vi "level_probe.vi"(5 "Run VI":bool, 6 "Set # of Turns Open (Man)":dbl, 7 "Target Level (Auto)":dbl format="%.2f", 8 "stop":bool, 9 "Mode":enum32{"AUTOMATIC", "MANUAL"}(radio)=enum."MANUAL", 10 "position":refnum<vi>, 11 "level":refnum<vi>) -> ()   [LabVIEW 2019]
uses:
  <vilib>/numeric/Random Number (Range) DBL.vi
  <vilib>/Utility/config.llb/Read Key (String).vi
  <vilib>/Utility/config.llb/Read Key (Path).vi
  <vilib>/Utility/file.llb/Read Delimited Spreadsheet (DBL).vi
  <vilib>/Utility/file.llb/Write Delimited Spreadsheet (DBL).vi
  subvi_motor/global_motor.vi
  <vilib>/addons/control/pid/NI_PID_autopid.lvlib
  <vilib>/Utility/config.llb/NI_LVConfig.lvlib
panel:
  out "read buffer":string
  in  "Mode 2":enum32{"Continuous", "Sample and Hold"}(radio)
  in  "Motor Enabled":bool=TRUE
  out "levelbuffer":string
  out "Level":dbl(slide) scale=0.0..100.0
  in  "Save PID gains":bool
  in  "Load PID gains":bool
  in  "Recalibrate":bool
  in  "Current Position":dbl
  out "Motor Connected":bool
  in  "Enable Advanced Controls":bool
  in  "Log Data?":bool
  out "maxsteps":dbl
  out "minsteps":dbl
  in  "Min Open (Auto)":dbl=0.25
  in  "Max Open (Auto)":dbl=0.75
  out "Level":dynamicdata(graph)
  out "Error":dynamicdata(graph)
  in  "PID gains":T1={"proportional gain (Kc)"=10.0, "integral time (Ti, min)"=0.002, "derivative time (Td, min)"=0.2} {"derivative time (Td, min)" format="%.3f"; "integral time (Ti, min)" format="%.3f"; "proportional gain (Kc)" format="%.3f"}
  out "Valve Position":dynamicdata(graph)
  out "# of Turns Open":dbl
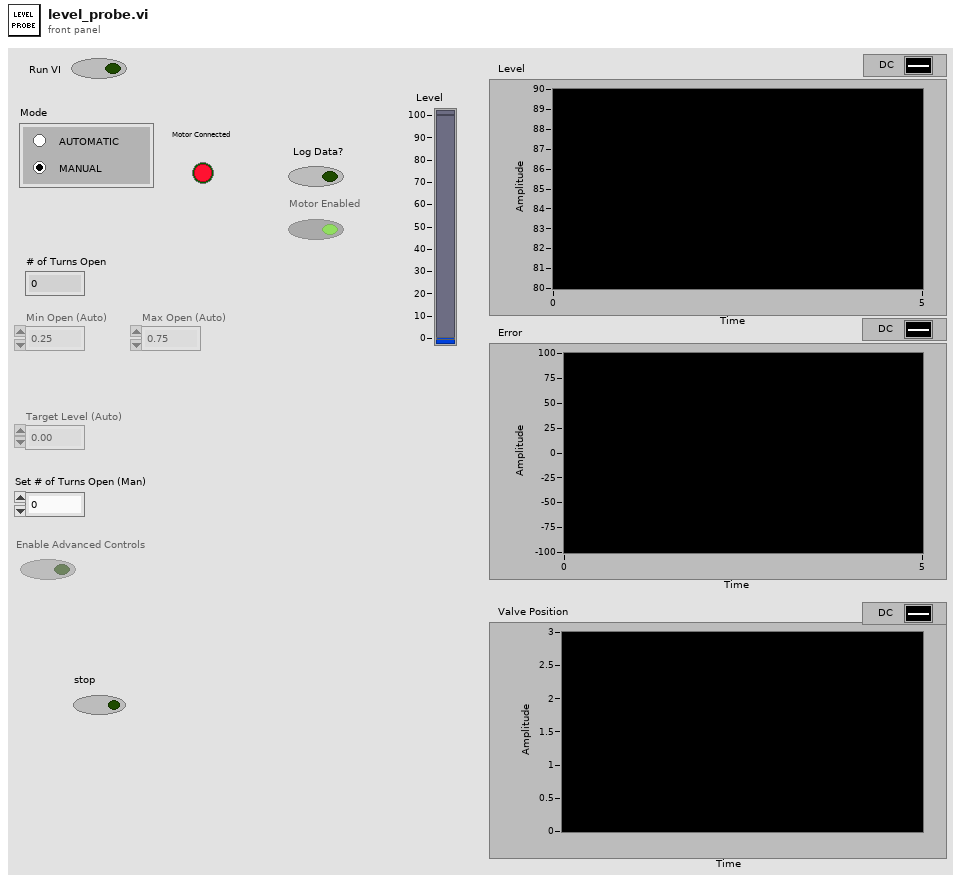
[diagram p1: front panel]
types:
  T1 = cluster{"proportional gain (Kc)":dbl, "integral time (Ti, min)":dbl, "derivative time (Td, min)":dbl}
  T2 = enum16{"open", "replace", "create", "open or create", "replace or create", "replace or create with confirmation"}
  T3 = enum8{"Enabled", "Disabled", "Disabled and Grayed Out"}
  T4 = typedef "NI_LVConfig.lvlib/Config Data RefNum.ctl" = refnum<k1>
  T5 = cluster{"first row[0]":dbl, "first row[1]":dbl, "first row[2]":dbl, "first row[3]":dbl, "first row[4]":dbl, "first row[5]":dbl, "first row[6]":dbl, "first row[7]":dbl, "first row[8]":dbl}
  T6 = cluster{"first row[0]":dbl, "first row[1]":dbl, "first row[2]":dbl}
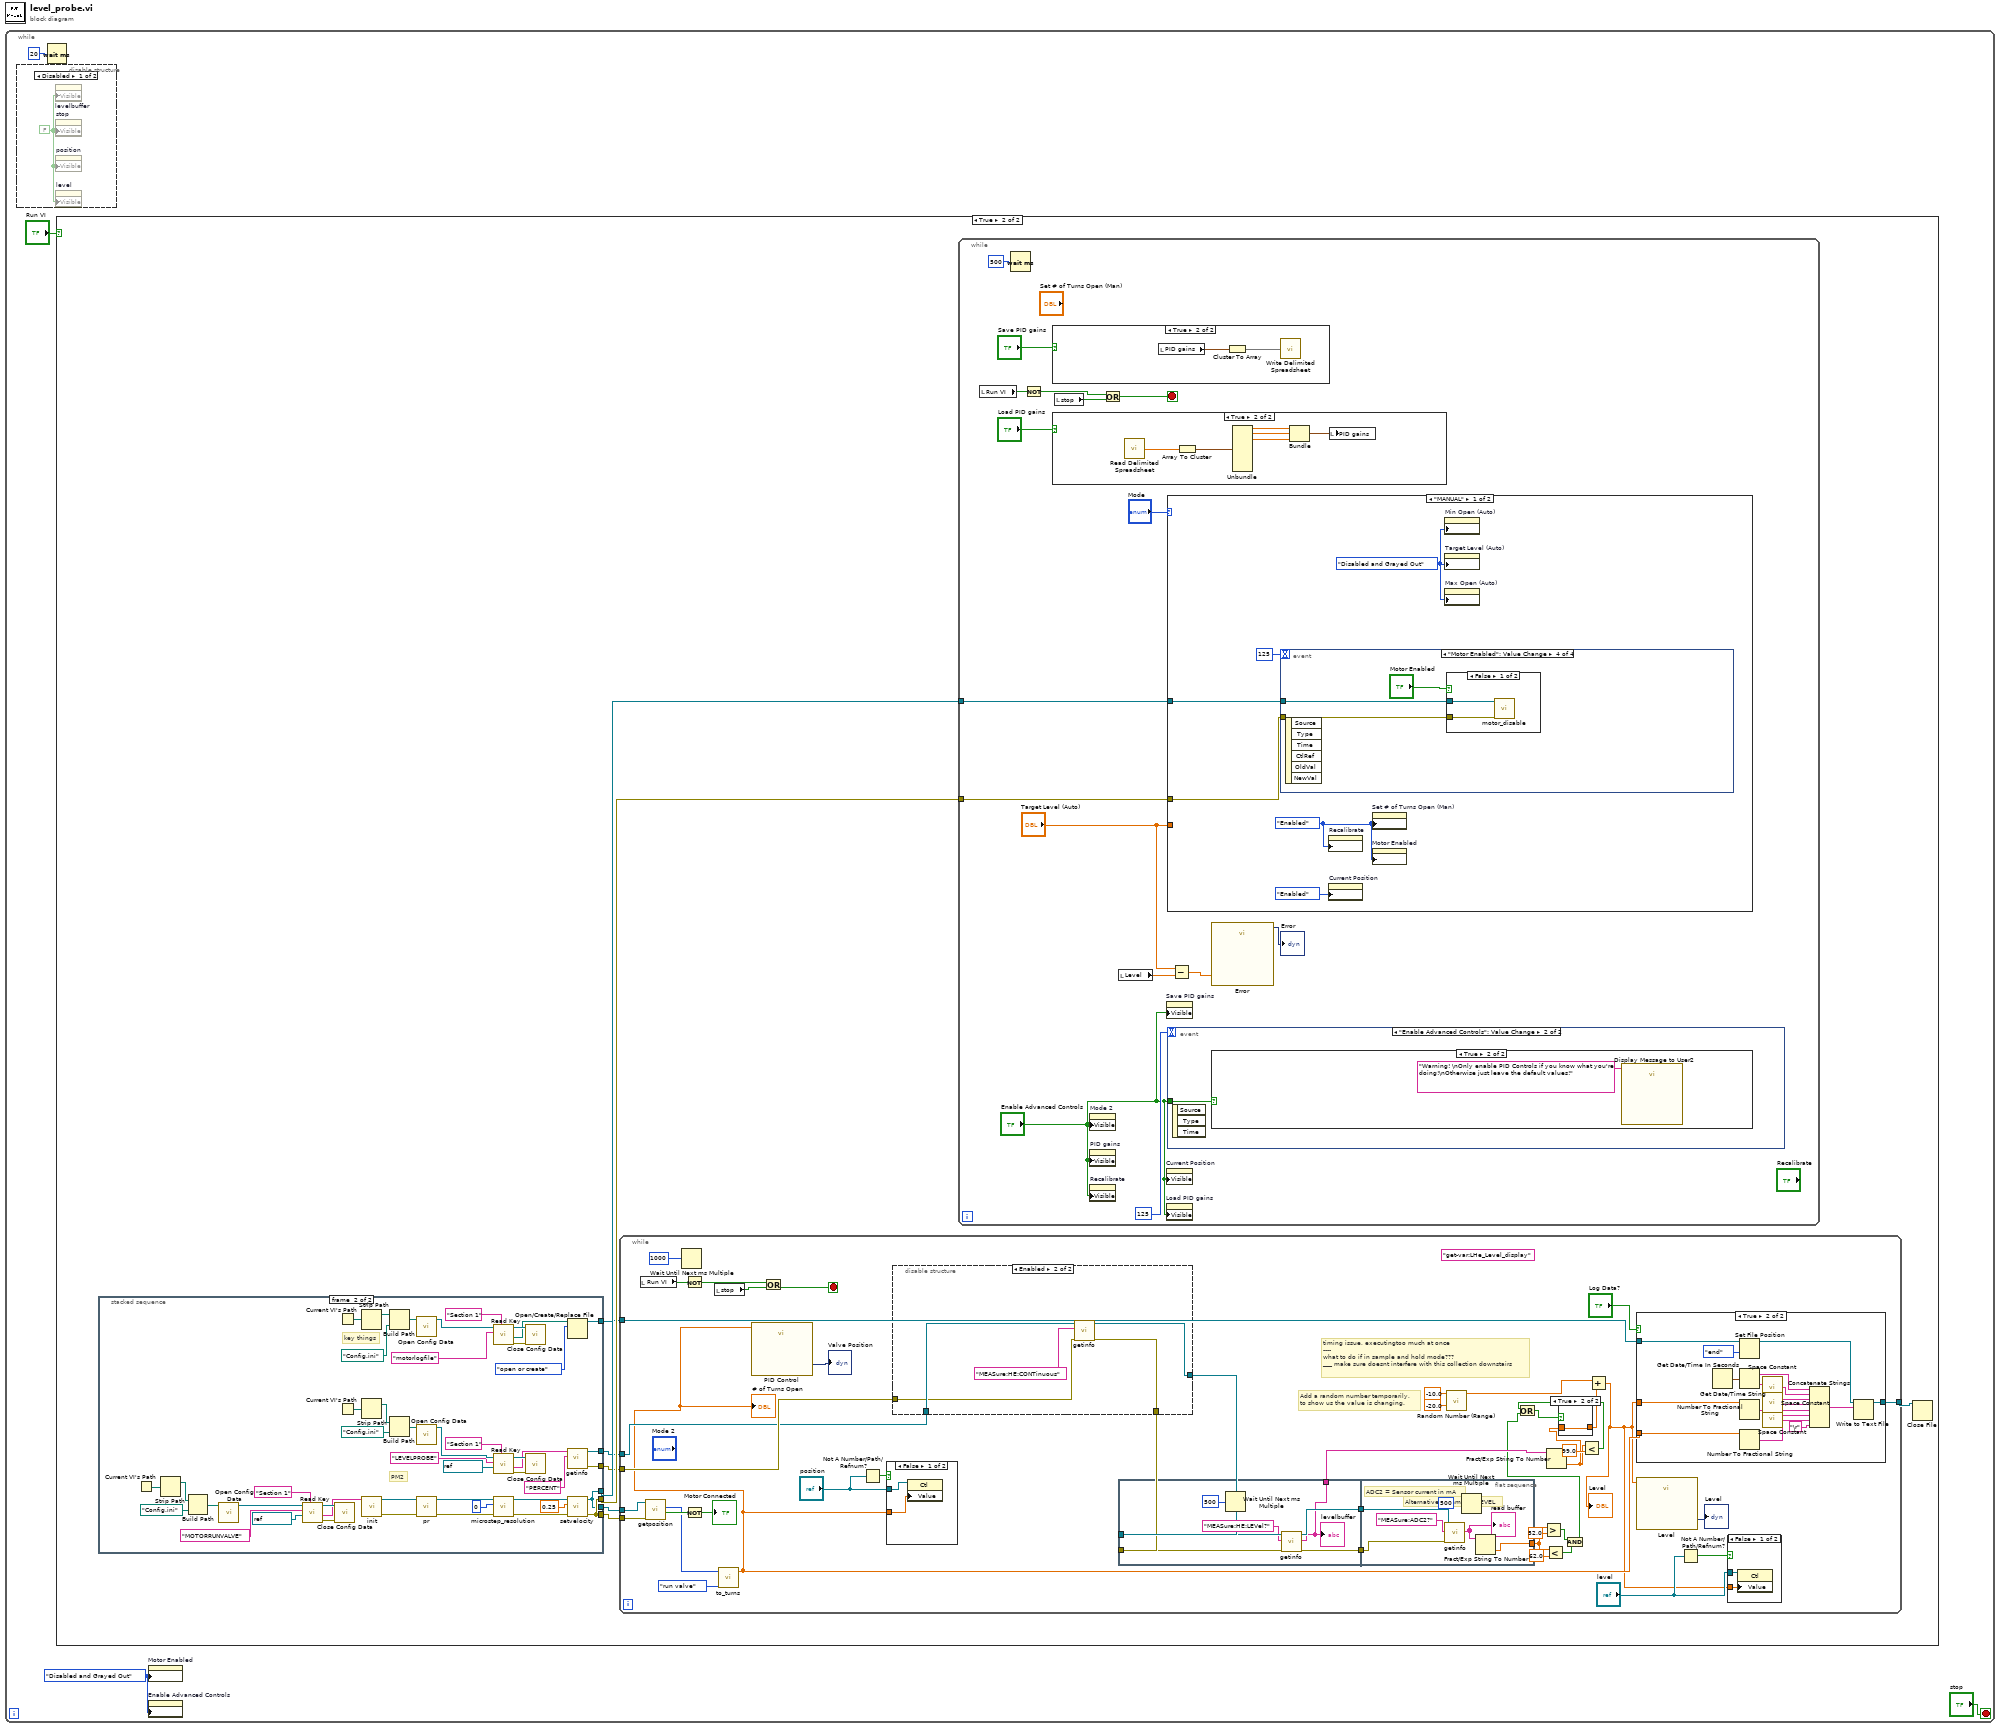
[diagram p0: block diagram]
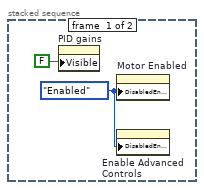
[diagram p4: hidden frame]
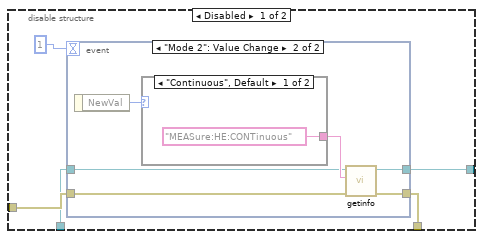
[diagram p5: hidden frame]
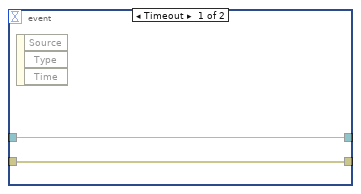
[diagram p6: hidden frame]
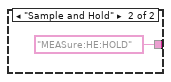
[diagram p7: hidden frame]
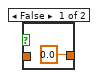
[diagram p10: hidden frame]
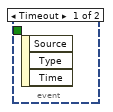
[diagram p12: hidden frame]
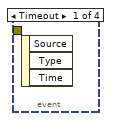
[diagram p16: hidden frame]
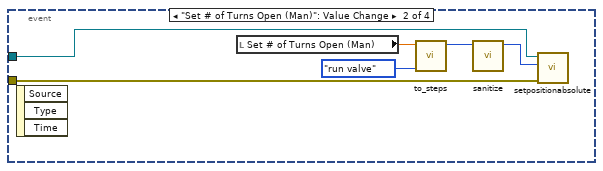
[diagram p17: hidden frame]
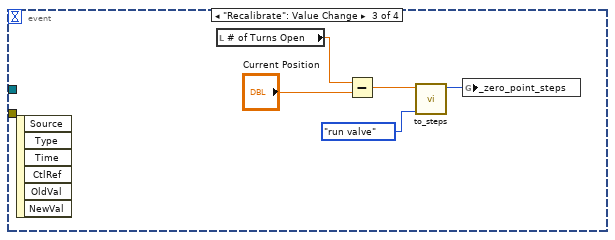
[diagram p18: hidden frame]
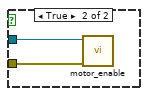
[diagram p19: hidden frame]
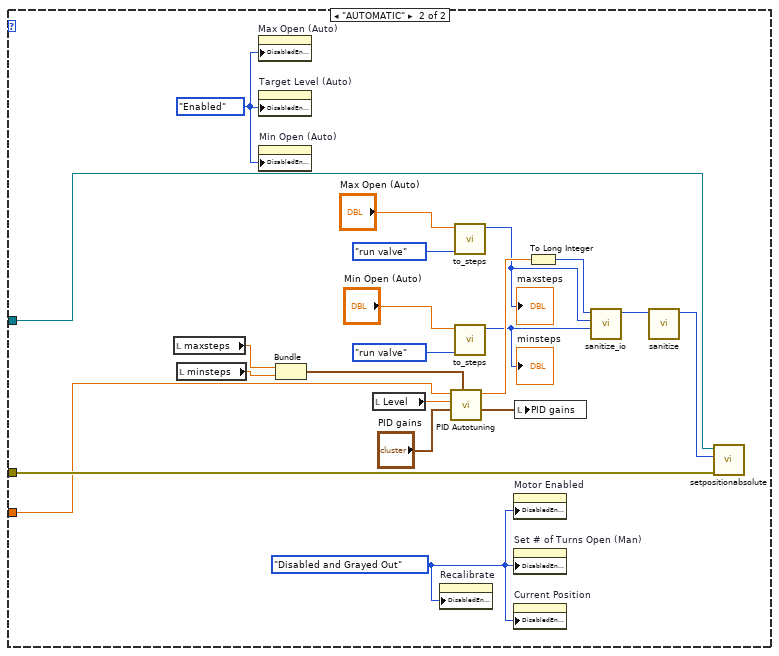
[diagram p20: hidden frame]
diagram:
  n1 = while {
    stop <- "stop" stop-if-true
    w1 = T3."Disabled and Grayed Out" ("Disabled")
    n2 = disable-structure shown="Disabled" {
      frame Disabled {
        w5 = FALSE ("Visible")
        n3 = property on="levelbuffer" class="Str"("Visible"=w5) -> ()  [unwired: 2 in, 2 out]
        n4 = property on="stop" class="Bool (strict)"("Visible"=w5) -> ()  [unwired: 2 in, 2 out]
        n5 = property on="position" class="LVObjRef (strict)"("Visible"=w5) -> ()  [unwired: 2 in, 2 out]
        n6 = property on="level" class="LVObjRef (strict)"("Visible"=w5) -> ()  [unwired: 2 in, 2 out]
      }
      frame Enabled {
      }
    }
    n7 = Wait (ms)(milliseconds to wait=u32 20) -> ()  [unwired: 1 out]
    n8 = case shown="True" "Run VI" {
      frame False {
      }
      frame True {
        n9 = stacked-sequence {
          tunnel: [_ w61] -> w13
          tunnel: [_ w61] -> w12
          tunnel: [_ w60] -> w11
          tunnel: [_ w60] -> w10
          tunnel: [_ w55] -> w9
          tunnel: [_ w54] -> w8
          tunnel: [_ w53] -> w7
          frame #0 {
            w14 = T3."Enabled" ("Disabled")
            n10 = property on="PID gains" class="Clust (strict)"("Visible"=FALSE) -> ()  [unwired: 2 in, 2 out]
            n11 = property on="Motor Enabled" class="Bool (strict)"("DisabledEnum"=w14) -> ()  [unwired: 2 in, 2 out]
            n12 = property on="Enable Advanced Controls" class="Bool (strict)"("DisabledEnum"=w14) -> ()  [unwired: 2 in, 2 out]
          }
          frame #1 {
            # "PM2"
            # "key things"
            n13 = Current VI's Path() -> (path=w39:path)
            n14 = Strip Path(path=w39) -> (stripped path=w38:path)  [unwired: 1 out]
            n15 = Build Path(base path=w38, name or relative path=path "Config.ini" ("default name")) -> (appended path=w42:path)
            n16 = call <vilib>:"Open Config Data.vi"("configuration file path"=w42) -> ("refnum"=w47:T4)  [unwired: 8 in, 2 out]
            n17 = call-poly <vilib>:"Read Key.vi"("section"="Section 1", "default value"=refnum<visa-resource-name> "COM5" ("VISA resource name"), "key"="MOTORRUNVALVE", "refnum"=w47) -> ("error out"=w41:errorcluster, "value"=w37:string, "refnum out"=w45:T4)  [unwired: 4 in, 1 out]
            n18 = call <vilib>:"Close Config Data.vi"("error in (no error)"=w41, "refnum"=w45) -> ()  [unwired: 8 in, 2 out]
            n19 = Current VI's Path() -> (path=w19:path)
            n20 = Current VI's Path() -> (path=w28:path)
            n21 = Strip Path(path=w19) -> (stripped path=w18:path)  [unwired: 1 out]
            n22 = Strip Path(path=w28) -> (stripped path=w27:path)  [unwired: 1 out]
            n23 = call "init.vi"("VISA resource name"=w37) -> ("error out"=w49:errorcluster, "VISA resource name 2"=w51:refnum<visa-resource-name>)  [unwired: 9 in]
            n24 = Build Path(base path=w18, name or relative path=path "Config.ini" ("default name")) -> (appended path=w21:path)
            n25 = Build Path(base path=w27, name or relative path=path "Config.ini" ("default name")) -> (appended path=w31:path)
            n26 = call <vilib>:"Open Config Data.vi"("configuration file path"=w21) -> ("refnum"=w26:T4)  [unwired: 8 in, 2 out]
            n27 = call <vilib>:"Open Config Data.vi"("configuration file path"=w31) -> ("refnum"=w36:T4)  [unwired: 8 in, 2 out]
            n28 = call "pr.vi"("error in (no error)"=w49, "VISA resource name"=w51) -> ("error out"=w48:errorcluster, "VISA resource name 2"=w50:refnum<visa-resource-name>)  [unwired: 8 in]
            n29 = call-poly <vilib>:"Read Key.vi"("section"="Section 1", "key"="motorlogfile", "refnum"=w26) -> ("error out"=w20:errorcluster, "value"=w17:path, "refnum out"=w24:T4)  [unwired: 5 in, 1 out]
            n30 = call-poly <vilib>:"Read Key.vi"("section"="Section 1", "default value"=refnum<visa-resource-name> "COM8" ("VISA resource name"), "key"="LEVELPROBE", "refnum"=w36) -> ("error out"=w30:errorcluster, "value"=w16:string, "refnum out"=w34:T4)  [unwired: 4 in, 1 out]
            n31 = call "microstep_resolution.vi"("error in (no error)"=w48, "number"=0, "VISA in"=w50) -> ("error out"=w58:errorcluster, "VISA out"=w57:refnum<visa-resource-name>)  [unwired: 7 in]
            n32 = call <vilib>:"Close Config Data.vi"("error in (no error)"=w20, "refnum"=w24) -> ()  [unwired: 8 in, 2 out]
            n33 = call <vilib>:"Close Config Data.vi"("error in (no error)"=w30, "refnum"=w34) -> ()  [unwired: 8 in, 2 out]
            n34 = Open/Create/Replace File(file path (use dialog)=w17, operation (0:open)=T2."open or create") -> (refnum out=w53:refnum<file>)  [unwired: 4 in, 2 out]
            n35 = call "getinfo.vi"("string"="PERCENT", "VISA resource name"=w16) -> ("error out"=w54:errorcluster, "VISA resource name 2"=w55:refnum<visa-resource-name>)  [unwired: 7 in, 1 out]
            n36 = call "setvelocity.vi"("error in (no error)"=w58, "Velocity"=0.25, "VISA in"=w57) -> ("error out"=w61:errorcluster, "VISA out"=w60:refnum<visa-resource-name>)  [unwired: 7 in]
          }
        }
        n37 = while {
          tunnel: w12 -> [w105]
          tunnel: w10 -> [w104]
          tunnel: w9 -> [w89]
          tunnel: w8 -> [w90]
          tunnel: w7 -> [w93]
          tunnel: [w92] -> w6
          stop <- w95 stop-if-true
          (unwired) "get-var:LHe_Level_display" ("string")
          # "Add a random number temporarily,\nto show us the value is changing."
          # "timing issue, executingtoo much at once\n----\nwhat to do if in sample and hold mode???\n___ make sure doesnt interfere with this collection downstairs"
          # "Alternative Command: LEVEL"
          n38 = local read "Run VI"() -> (w97:bool)
          n39 = call "getposition.vi"("error in (no error)"=w105, "VISA resource name"=w104) -> ("Is Null?"=w100:bool, "Position"=w98:i32)  [unwired: 6 in, 2 out]
          n40 = Wait Until Next ms Multiple(millisecond multiple=u32 1000 ("milliseconds to wait")) -> ()  [unwired: 1 out]
          n41 = Not(x=w97) -> (.not. x?=w96:bool)
          n42 = Not(x=w100) -> (.not. x?=→"Motor Connected":bool)
          n43 = local read "stop"() -> (w94:bool)
          n44 = call "to_turns.vi"("Radio Buttons"=enum32{"run valve", "bypass valve"}."run valve", "Steps"=w98) -> ("Turns"=w71:dbl)  [unwired: 9 in]
          "# of Turns Open" <- w71
          n45 = call "PID Control"("Offset"=w71) -> ("DC"=→"Valve Position":dynamicdata)  [unwired: 13 in, 1 out]
          n46 = Or(x=w96, y=w94) -> (x .or. y?=w95:bool)
          n47 = Not A Number/Path/Refnum?(number/path/refnum="position") -> (NaN/Path/Refnum?=w70:bool)
          n48 = case shown="False" w70 {
            tunnel: "position" -> [w129 _]
            tunnel: w71 -> [w128 _]
            frame False {
              n49 = property class="Ctl"(reference=w129, "Value"=w128) -> ()  [unwired: 1 in, 2 out]
            }
            frame True {
            }
          }
          n50 = disable-structure shown="Enabled" {
            disable-tunnel: w90 -> [w109 w123]
            disable-tunnel: w89 -> [w108 w124]
            disable-tunnel: [w107 w121] -> w88
            disable-tunnel: [w106 w122] -> w87
            frame Disabled {
              n51 = event shown="[1] \"Mode 2\": Value Change" {
                selector: _ -> [_ _]
                dyn-events: _ -> [_ _]
                timeout: 1 -> [_ _]
                tunnel: w109 -> [w111 w115]
                tunnel: w108 -> [w112 w116]
                tunnel: [w112 w114] -> w107
                tunnel: [w111 w113] -> w106
                event Timeout {
                  n52 = event-data() -> ()  [unwired: 1 in, 3 out]
                }
                event "Mode 2": Value Change {
                  n53 = event-data() -> ("NewVal"=w118:enum32{"Continuous", "Sample and Hold"})  [unwired: 1 in]
                  n54 = case shown="\"Continuous\", Default" w118 {
                    tunnel: ["MEASure:HE:CONTinuous" ("string") "MEASure:HE:HOLD"] -> w117
                    frame "Continuous", Default {
                    }
                    frame "Sample and Hold" {
                    }
                  }
                  n55 = call "getinfo.vi"("error in (no error)"=w115, "string"=w117, "VISA resource name"=w116) -> ("error out"=w113:errorcluster, "VISA resource name 2"=w114:refnum<visa-resource-name>)  [unwired: 6 in, 1 out]
                }
              }
            }
            frame Enabled {
              n56 = call "getinfo.vi"("error in (no error)"=w123, "string"="MEASure:HE:CONTinuous", "VISA resource name"=w124) -> ("error out"=w122:errorcluster, "VISA resource name 2"=w121:refnum<visa-resource-name>)  [unwired: 6 in, 1 out]
            }
          }
          n57 = flat-sequence {
            tunnel: w88 -> [w138]
            tunnel: w87 -> [w136]
            tunnel: [w134] -> w85
            tunnel: [w133] -> w84
            tunnel: [w132] -> w83
            tunnel: w85 -> [w143]
            tunnel: w84 -> [w142]
            tunnel: [w139] -> w81
            frame #0 {
              n58 = Wait Until Next ms Multiple(millisecond multiple=u32 500) -> ()  [unwired: 1 out]
              n59 = call "getinfo.vi"("error in (no error)"=w136, "string"="MEASure:HE:LEVel?", "VISA resource name"=w138) -> ("error out"=w133:errorcluster, "read buffer"=w132:string, "VISA resource name 2"=w134:refnum<visa-resource-name>)  [unwired: 6 in]
              "levelbuffer" <- w132
            }
            frame #1 {
              # "ADC2 = Sensor current in mA"
              n60 = call "getinfo.vi"("error in (no error)"=w142, "string"="MEASure:ADC2?", "VISA resource name"=w143) -> ("read buffer"=w140:string)  [unwired: 6 in, 2 out]
              "read buffer" <- w140
              n61 = Wait Until Next ms Multiple(millisecond multiple=u32 500) -> ()  [unwired: 1 out]
              n62 = Fract/Exp String To Number(string=w140) -> (number=w139:dbl)  [unwired: 3 in, 1 out]
            }
          }
          n63 = call-poly <vilib>:"Random Number (Range).vi"("lower bound (0)"=-20.0, "upper bound (100)"=-10.0) -> ("number"=w63:dbl)  [unwired: 9 in]
          n64 = Greater?(x=w81, y=52.0) -> (0:w79:bool)
          n65 = Less?(x=w81, y=62.0) -> (x < y?=w78:bool)
          n66 = Fract/Exp String To Number(string=w83) -> (number=w74:dbl)  [unwired: 3 in, 1 out]
          n67 = And(x=w79, y=w78) -> (x .and. y?=w75:bool)
          n68 = Less?(x=w74, y=99.0) -> (x < y?=w76:bool)
          n69 = Or(x=w76, y=w75) -> (x .or. y?=w73:bool)
          n70 = case shown="True" w73 {
            tunnel: [0.0 w131] -> w67
            tunnel: w74 -> [_ w131]
            frame False {
            }
            frame True {
            }
          }
          n71 = Add(x=w63, y=w67) -> (x+y=w66:dbl)
          "Level" <- w66
          n72 = case shown="True" "Log Data?" {
            tunnel: w71 -> [_ w161]
            tunnel: w66 -> [_ w156]
            tunnel: w93 -> [w145 w151]
            tunnel: [w145 w150] -> w92
            frame False {
            }
            frame True {
              n73 = Get Date/Time In Seconds() -> (seconds since 1Jan1904=w149:timestamp)
              n74 = Set File Position(refnum=w151, from (0:start)=enum16{"start", "end", "current"}."end") -> (refnum out=w157:refnum<file>)  [unwired: 2 in, 1 out]
              n75 = Get Date/Time String(seconds (now)=w149) -> (date string=w147:string, time string=w148:string)  [unwired: 2 in]
              n76 = Number To Fractional String(number=w156) -> (F-format string=w155:string)  [unwired: 3 in]
              n77 = Number To Fractional String(number=w161) -> (F-format string=w153:string)  [unwired: 3 in]
              n78 = call <vilib>:"Space Constant.vi"() -> ("String"=w146:string)
              n79 = call <vilib>:"Space Constant.vi"() -> ("String"=w159:string)
              n80 = call <vilib>:"Space Constant.vi"() -> ("String"=w154:string)
              n81 = Concatenate Strings(w147, w146, w148, w159, w155, w154, w153, "\r") -> (w160:string)
              n82 = Write to Text File(file (use dialog)=w157, text=w160) -> (refnum out=w150:refnum<file>)  [unwired: 2 in, 2 out]
            }
          }
          n83 = call "Level"("Offset"=w66) -> ("DC"=→"Level":dynamicdata)  [unwired: 13 in, 1 out]
          n84 = Not A Number/Path/Refnum?(number/path/refnum="level") -> (NaN/Path/Refnum?=w68:bool)
          n85 = case shown="False" w68 {
            tunnel: "level" -> [w127 _]
            tunnel: w66 -> [w126 _]
            frame False {
              n86 = property class="Ctl"(reference=w127, "Value"=w126) -> ()  [unwired: 1 in, 2 out]
            }
            frame True {
            }
          }
        }
        n87 = while {
          tunnel: w13 -> [w176]
          tunnel: w11 -> [w175]
          stop <- w164 stop-if-true
          n88 = local read "Run VI"() -> (w167:bool)
          n89 = Wait (ms)(milliseconds to wait=u32 500) -> ()  [unwired: 1 out]
          n90 = Not(x=w167) -> (.not. x?=w165:bool)
          n91 = case shown="True" "Save PID gains" {
            frame False {
            }
            frame True {
              n92 = local read "PID gains"() -> (w181:T1)
              n93 = Cluster To Array(cluster=w181) -> (array=w180:dbl[])
              n94 = call-poly <vilib>:"Write Delimited Spreadsheet.vi"("1D data"=w180) -> ()  [unwired: 13 in, 2 out]
            }
          }
          n95 = case shown="True" "Load PID gains" {
            frame False {
            }
            frame True {
              n96 = call-poly <vilib>:"Read Delimited Spreadsheet.vi"() -> ("first row"=w187:dbl[])  [unwired: 10 in, 5 out]
              n97 = Array To Cluster(array=w187) -> (cluster=w186:T5)
              n98 = Unbundle(w186) -> ("first row[0]"=w185:dbl, "first row[1]"=w184:dbl, "first row[2]"=w183:dbl)  [unwired: 6 out]
              n99 = Bundle("first row[0]"=w185, "first row[1]"=w184, "first row[2]"=w183) -> (w182:T6)  [unwired: 1 in]
              n100 = local write "PID gains"(w182) -> ()
            }
          }
          n101 = local read "stop"() -> (w163:bool)
          n102 = property on="Mode 2" class="RadioBtnsControl (strict)"("Visible"="Enable Advanced Controls") -> ()  [unwired: 2 in, 2 out]
          n103 = property on="PID gains" class="Clust (strict)"("Visible"="Enable Advanced Controls") -> ()  [unwired: 2 in, 2 out]
          n104 = property on="Recalibrate" class="Bool"("Visible"="Enable Advanced Controls") -> ()  [unwired: 2 in, 2 out]
          n105 = Or(x=w165, y=w163) -> (x .or. y?=w164:bool)
          n106 = local read "Level"() -> (w166:dbl)
          n107 = property on="Save PID gains" class="Bool"("Visible"="Enable Advanced Controls") -> ()  [unwired: 2 in, 2 out]
          n108 = property on="Current Position" class="DigNum (strict)"("Visible"="Enable Advanced Controls") -> ()  [unwired: 2 in, 2 out]
          n109 = property on="Load PID gains" class="Bool"("Visible"="Enable Advanced Controls") -> ()  [unwired: 2 in, 2 out]
          n110 = case shown="\"MANUAL\"" "Mode" {
            tunnel: w175 -> [w193 w229]
            tunnel: w176 -> [w192 w230]
            tunnel: "Target Level (Auto)" -> [_ w228]
            frame "MANUAL" {
              w189 = T3."Enabled" ("Disabled")
              w188 = T3."Disabled and Grayed Out" ("Disabled")
              n111 = event shown="[3] \"Motor Enabled\": Value Change" {
                selector: _ -> [_ _ _ _]
                dyn-events: _ -> [_ _ _ _]
                timeout: 125 -> [_ _ _ _]
                tunnel: w193 -> [_ w198 _ w207]
                tunnel: w192 -> [_ w197 _ w206]
                event Timeout {
                  n112 = event-data() -> ()  [unwired: 1 in, 3 out]
                }
                event "Set # of Turns Open (Man)": Value Change {
                  n113 = event-data() -> ()  [unwired: 1 in, 3 out]
                  n114 = local read "Set # of Turns Open (Man)"() -> (w196:dbl)
                  n115 = call "to_steps.vi"("Radio Buttons"=enum32{"run valve", "bypass valve"}."run valve", "Turns"=w196) -> ("Steps"=w195:i32)  [unwired: 9 in]
                  n116 = call "sanitize.vi"("Input"=w195) -> ("Sanitized Input"=w199:i32)  [unwired: 10 in]
                  n117 = call "setpositionabsolute.vi"("error in (no error)"=w197, "Position Aboslute"=w199, "VISA in"=w198) -> ()  [unwired: 7 in, 2 out]
                }
                event "Recalibrate": Value Change {
                  n118 = event-data() -> ()  [unwired: 1 in, 6 out]
                  n119 = local read "# of Turns Open"() -> (w202:dbl)
                  n120 = Subtract(x=w202, y="Current Position") -> (x-y=w203:dbl)
                  n121 = call "to_steps.vi"("Radio Buttons"=enum32{"run valve", "bypass valve"}."run valve", "Turns"=w203) -> ("Steps"=w204:i32)  [unwired: 9 in]
                  n122 = global write "global_motor.vi" "_zero_point_steps"(w204) -> ()
                }
                event "Motor Enabled": Value Change {
                  n123 = event-data() -> ()  [unwired: 1 in, 6 out]
                  n124 = case shown="False" "Motor Enabled" {
                    tunnel: w207 -> [w208 w211]
                    tunnel: w206 -> [w209 w210]
                    frame False {
                      n125 = call "motor_disable.vi"("error in (no error)"=w209, "VISA resource name"=w208) -> ()  [unwired: 8 in, 2 out]
                    }
                    frame True {
                      n126 = call "motor_enable.vi"("error in (no error)"=w210, "VISA resource name"=w211) -> ()  [unwired: 8 in, 2 out]
                    }
                  }
                }
              }
              n127 = property on="Recalibrate" class="Bool"("DisabledEnum"=w189) -> ()  [unwired: 2 in, 2 out]
              n128 = property on="Current Position" class="DigNum (strict)"("DisabledEnum"=T3."Enabled" ("Disabled")) -> ()  [unwired: 2 in, 2 out]
              n129 = property on="Set # of Turns Open (Man)" class="DigNum (strict)"("DisabledEnum"=w189) -> ()  [unwired: 2 in, 2 out]
              n130 = property on="Motor Enabled" class="Bool (strict)"("DisabledEnum"=w189) -> ()  [unwired: 2 in, 2 out]
              n131 = property on="Min Open (Auto)" class="DigNum (strict)"("DisabledEnum"=w188) -> ()  [unwired: 2 in, 2 out]
              n132 = property on="Target Level (Auto)" class="DigNum (strict)"("DisabledEnum"=w188) -> ()  [unwired: 2 in, 2 out]
              n133 = property on="Max Open (Auto)" class="DigNum (strict)"("DisabledEnum"=w188) -> ()  [unwired: 2 in, 2 out]
            }
            frame "AUTOMATIC" {
              w215 = T3."Disabled and Grayed Out" ("Disabled")
              w214 = T3."Enabled" ("Disabled")
              n134 = local read "maxsteps"() -> (w227:dbl)
              n135 = local read "minsteps"() -> (w226:dbl)
              n136 = property on="Max Open (Auto)" class="DigNum (strict)"("DisabledEnum"=w214) -> ()  [unwired: 2 in, 2 out]
              n137 = property on="Target Level (Auto)" class="DigNum (strict)"("DisabledEnum"=w214) -> ()  [unwired: 2 in, 2 out]
              n138 = property on="Min Open (Auto)" class="DigNum (strict)"("DisabledEnum"=w214) -> ()  [unwired: 2 in, 2 out]
              n139 = Bundle("maxsteps"=w227, "minsteps"=w226) -> (w220:cluster{"maxsteps":dbl, "minsteps":dbl})  [unwired: 1 in]
              n140 = local read "Level"() -> (w216:dbl)
              n141 = property on="Recalibrate" class="Bool"("DisabledEnum"=w215) -> ()  [unwired: 2 in, 2 out]
              n142 = call <vilib>:"PID Autotuning.vi"("output range"=w220, "PID gains"="PID gains", "process variable"=w216, "setpoint"=w228) -> ("PID gains out"=w219:T1, "output"=w231:dbl)  [unwired: 4 in, 2 out]
              n143 = call "to_steps.vi"("Radio Buttons"=enum32{"run valve", "bypass valve"}."run valve", "Turns"="Max Open (Auto)") -> ("Steps"=w222:i32)  [unwired: 9 in]
              "maxsteps" <- w222
              n144 = call "to_steps.vi"("Radio Buttons"=enum32{"run valve", "bypass valve"}."run valve", "Turns"="Min Open (Auto)") -> ("Steps"=w221:i32)  [unwired: 9 in]
              "minsteps" <- w221
              n145 = property on="Motor Enabled" class="Bool (strict)"("DisabledEnum"=w215) -> ()  [unwired: 2 in, 2 out]
              n146 = property on="Set # of Turns Open (Man)" class="DigNum (strict)"("DisabledEnum"=w215) -> ()  [unwired: 2 in, 2 out]
              n147 = property on="Current Position" class="DigNum (strict)"("DisabledEnum"=w215) -> ()  [unwired: 2 in, 2 out]
              n148 = local write "PID gains"(w219) -> ()
              n149 = To Long Integer(number=w231) -> (32bit integer=w225:i32)
              n150 = call "sanitize_io.vi"("min"=w221, "max"=w222, "Input"=w225) -> ("Sanitized Input"=w217:i32)  [unwired: 8 in]
              n151 = call "sanitize.vi"("Input"=w217) -> ("Sanitized Input"=w218:i32)  [unwired: 10 in]
              n152 = call "setpositionabsolute.vi"("error in (no error)"=w230, "Position Aboslute"=w218, "VISA in"=w229) -> ()  [unwired: 7 in, 2 out]
            }
          }
          n153 = event shown="[1] \"Enable Advanced Controls\": Value Change" {
            selector: _ -> [_ _]
            dyn-events: _ -> [_ _]
            timeout: 125 -> [_ _]
            tunnel: "Enable Advanced Controls" -> [_ w178]
            event Timeout {
              n154 = event-data() -> ()  [unwired: 1 in, 3 out]
            }
            event "Enable Advanced Controls": Value Change {
              n155 = event-data() -> ()  [unwired: 1 in, 3 out]
              n156 = case shown="True" w178 {
                frame False {
                }
                frame True {
                  n157 = call "Display Message to User2"("Message"="Warning! \nOnly enable PID Controls if you know what you're doing!\nOtherwise just leave the default values!") -> ()  [unwired: 9 in, 2 out]
                }
              }
            }
          }
          n158 = Subtract(x="Target Level (Auto)", y=w166) -> (x-y=w172:dbl)
          n159 = call "Error"("Offset"=w172) -> ("DC"=→"Error":dynamicdata)  [unwired: 13 in, 1 out]
        }
        n160 = Close File(refnum=w6) -> ()  [unwired: 1 in, 2 out]
      }
    }
    n161 = property on="Motor Enabled" class="Bool (strict)"("DisabledEnum"=w1) -> ()  [unwired: 2 in, 2 out]
    n162 = property on="Enable Advanced Controls" class="Bool (strict)"("DisabledEnum"=w1) -> ()  [unwired: 2 in, 2 out]
  }
